vi "DVD Screensaver.vi"() -> ()   [LabVIEW 2018]
uses:
  <vilib>/Utility/miscctls.llb/LVPositionTypeDef.ctl
panel:
  out "DVD Video":bool
  in  "stop":bool
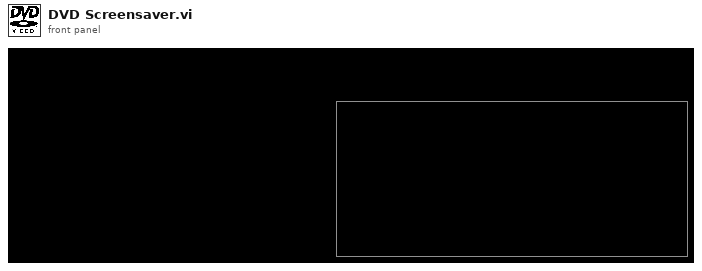
[diagram p1: front panel]
types:
  T1 = typedef "LVPositionTypeDef.ctl" = cluster{"Left":i32, "Top":i32}
  T2 = typedef "LVRectTypeDef.ctl" = cluster{"Left":i16, "Top":i16, "Right":i16, "Bottom":i16}
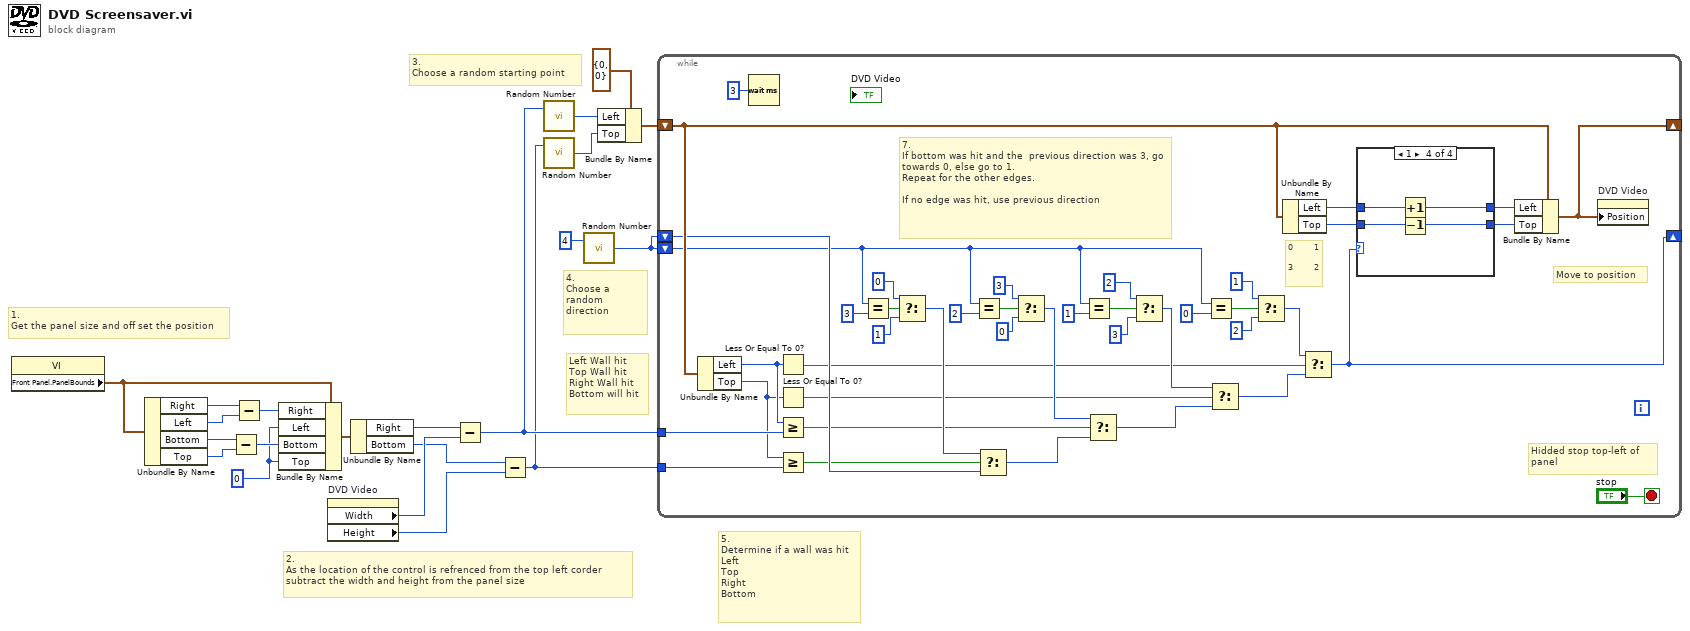
[diagram p0: block diagram]
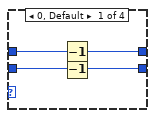
[diagram p2: hidden frame]
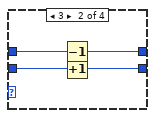
[diagram p3: hidden frame]
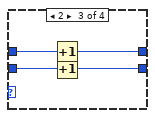
[diagram p4: hidden frame]
diagram:
  w13 = i16 0 ("Left")
  # "2.\nAs the location of the control is refrenced from the top left corder\nsubtract the width and height from the panel size"
  # "5.\nDetermine if a wall was hit\nLeft\nTop\nRight\nBottom"
  # "4.\nChoose a random direction"
  # "3.\nChoose a random starting point"
  # "1.\nGet the panel size and off set the position"
  # "Left Wall hit\nTop Wall hit\nRight Wall hit\nBottom will hit"
  n1 = property on="Property Node" class="VI"() -> ("Front Panel.PanelBounds"=w20:T2)  [unwired: 2 in, 2 out]
  n2 = Unbundle By Name(w20) -> ("Right"=w19:i16, "Left"=w18:i16, "Bottom"=w15:i16, "Top"=w14:i16)
  n3 = Subtract(x=w15, y=w14) -> (x-y=w16:i16)
  n4 = Subtract(x=w19, y=w18) -> (x-y=w17:i16)
  n5 = Bundle By Name(cluster=w20, "Right"=w17, "Left"=w13, "Bottom"=w16, "Top"=w13) -> (w12:T2)
  n6 = property on="DVD Video" class="Bool (strict)"() -> ("Width"=w10:u32, "Height"=w8:u32)  [unwired: 2 in, 2 out]
  n7 = Unbundle By Name(w12) -> ("Right"=w11:i16, "Bottom"=w9:i16)
  n8 = Subtract(x=w11, y=w10) -> (x-y=w6:u32)
  n9 = Subtract(x=w9, y=w8) -> (x-y=w5:u32)
  n10 = call "Random Number.vi"("Max"=w6) -> ("Out"=w3:u32)  [unwired: 2 in]
  n11 = call "Random Number.vi"("Max"=w5) -> ("Out"=w2:u32)  [unwired: 2 in]
  n12 = call "Random Number.vi"("Max"=4 ("t")) -> ("Out"=w1:u32)  [unwired: 2 in]
  n13 = Bundle By Name(cluster=T1 {"Left"=0, "Top"=0} ("Position"), "Left"=w3, "Top"=w2) -> (w7:T1)
  n14 = while {
    shift-right: [w59] -> _
    shift-left: w7 -> [w28]
    tunnel: w6 -> [w58]
    tunnel: w5 -> [w57]
    shift-right: [w30] -> _
    shift-left: w1 -> [w26]
    shift-left: w1 -> [w27]
    stop <- "stop" stop-if-true
    # "7.\nIf bottom was hit and the  previous direction was 3, go towards 0, else go to 1.\nRepeat for the other edges.\n\nIf no edge was hit, use previous direction"
    # "Move to position"
    # "Hidded stop top-left of \npanel"
    # "0       1\n\n3       2"
    n15 = Unbundle By Name(w28) -> ("Left"=w53:i32, "Top"=w52:i32)
    n16 = Wait (ms)(milliseconds to wait=u32 3) -> ()  [unwired: 1 out]
    n17 = Less Or Equal To 0?(x=w53) -> (x <= 0?=w25:bool)
    n18 = Less Or Equal To 0?(x=w52) -> (x <= 0?=w24:bool)
    n19 = Greater Or Equal?(x=w53, y=w58) -> (x >= y?=w23:bool)
    n20 = Greater Or Equal?(x=w52, y=w57) -> (x >= y?=w22:bool)
    n21 = Equal?(x=w26, y=3 ("t")) -> (x = y?=w37:bool)
    n22 = Select(t=0, s=w37, f=1) -> (s? t:f=w36:i32)
    n23 = Equal?(x=w26, y=2 ("t")) -> (x = y?=w45:bool)
    n24 = Select(t=w36, s=w22, f=w27) -> (s? t:f=w54:u32)
    n25 = Select(t=3, s=w45, f=0) -> (s? t:f=w40:i32)
    n26 = Equal?(x=w26, y=1 ("t")) -> (x = y?=w46:bool)
    n27 = Select(t=w40, s=w23, f=w54) -> (s? t:f=w55:u32)
    n28 = Select(t=2, s=w46, f=3) -> (s? t:f=w41:i32)
    n29 = Equal?(x=w26, y=0 ("t")) -> (x = y?=w51:bool)
    n30 = Select(t=w41, s=w24, f=w55) -> (s? t:f=w56:u32)
    n31 = Select(t=1, s=w51, f=2) -> (s? t:f=w48:i32)
    n32 = Unbundle By Name(w28) -> ("Left"=w63:i32, "Top"=w62:i32)
    n33 = Select(t=w48, s=w25, f=w56) -> (s? t:f=w30:u32)
    n34 = case shown="1" w30 {
      tunnel: w63 -> [w67 w71 w75 w79]
      tunnel: w62 -> [w66 w70 w74 w78]
      tunnel: [w65 w69 w73 w77] -> w61
      tunnel: [w64 w68 w72 w76] -> w60
      frame 0, Default {
        n35 = Decrement(x=w67) -> (x-1=w65:i32)
        n36 = Decrement(x=w66) -> (x-1=w64:i32)
      }
      frame 3 {
        n37 = Decrement(x=w71) -> (x-1=w69:i32)
        n38 = Increment(x=w70) -> (x+1=w68:i32)
      }
      frame 2 {
        n39 = Increment(x=w75) -> (x+1=w73:i32)
        n40 = Increment(x=w74) -> (x+1=w72:i32)
      }
      frame 1 {
        n41 = Increment(x=w79) -> (x+1=w77:i32)
        n42 = Decrement(x=w78) -> (x-1=w76:i32)
      }
    }
    n43 = Bundle By Name(cluster=w28, "Left"=w61, "Top"=w60) -> (w59:T1)
    n44 = property on="DVD Video" class="Bool (strict)"("Position"=w59) -> ()  [unwired: 2 in, 2 out]
  }
